vi "INI_bk9201.vi"(5 "MCListbox Ref":refnum<vi>, 9 "MCList Box Row":u8=3 max=8, 11 "Device INI Config File Path":path=path "D:/LABVIEW/Examples/INI Devices/DeviceConfig.ini") -> (0 "error out":errorcluster, 3 "Serial_VISA":T1)   [LabVIEW 2018]
uses:
  Examples - 32bit/SEQUENCER/SEQUENSER v10/Sequencer v10/Ctl/Serial_VISA.ctl
  <vilib>/Utility/miscctls.llb/LVRowAndColumnTypeDef.ctl
  <vilib>/Utility/config.llb/Read Key (String).vi
  <vilib>/Utility/config.llb/NI_LVConfig.lvlib
  <instrlib>/BK Precision 9200 Series/BK Precision 9200 Series.lvlib
panel:
  out "PowSupplay array":string[](array[string])
  out "PowSupply Read Buffer":string
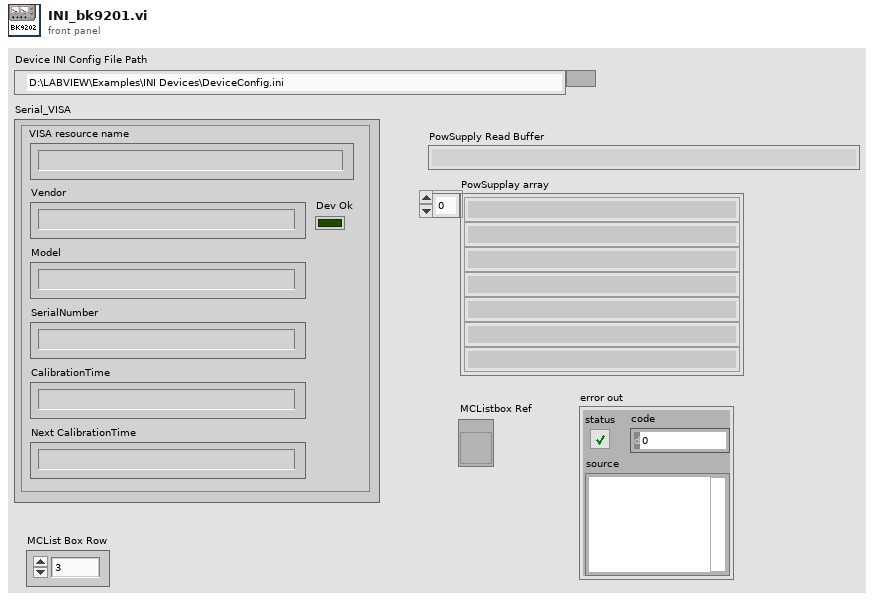
[diagram p1: front panel]
types:
  T1 = typedef "Serial_VISA.ctl" = cluster{"VISA resource name":string, "Vendor":string, "SerialNumber":string, "CalibrationTime":string, "Dev Ok":bool, "Model":string, "Next CalibrationTime":string}
  T2 = typedef "LVRowAndColumnTypeDef.ctl" = cluster{"Row":i32, "Column":i32}
  T3 = typedef "NI_LVConfig.lvlib/Config Data RefNum.ctl" = refnum<k1>
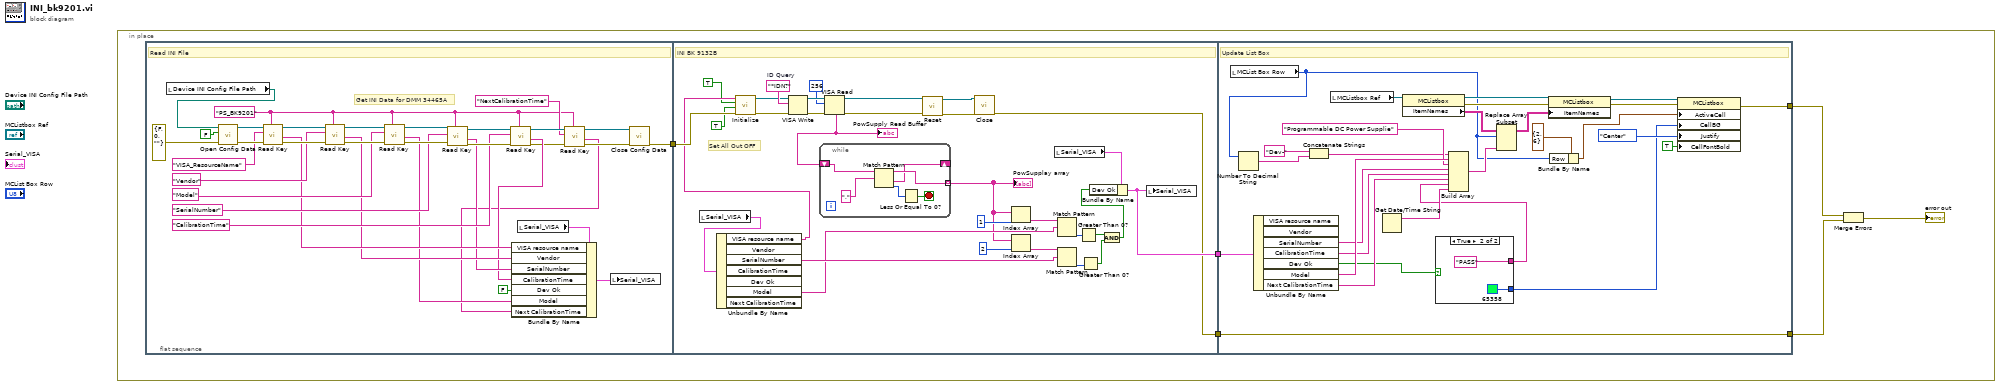
[diagram p0: block diagram]
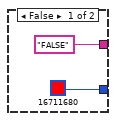
[diagram p2: hidden frame]
diagram:
  n1 = in-place {
    n2 = flat-sequence {
      tunnel: [w9] -> w6
      tunnel: w6 -> [w51]
      tunnel: [w42] -> w4
      tunnel: [w53] -> w1
      tunnel: [w85] -> w5
      tunnel: [w84] -> w3
      tunnel: w4 -> [w84]
      tunnel: w1 -> [w82]
      frame #0 {
        w13 = "PS_BK9201" ("section")
        # "Get INI Data for DMM 34465A"
        # "Read INI File"
        n3 = local read "Device INI Config File Path"() -> (w11:path)
        n4 = call <vilib>:"Open Config Data.vi"("error in (no error)"=errorcluster {"status"=FALSE, "code"=0, "source"=""} ("error constant"), "create file if necessary (T)"=FALSE, "configuration file path"=w11) -> ("error out"=w38:errorcluster, "refnum"=w39:T3)  [unwired: 6 in, 1 out]
        n5 = call-poly <vilib>:"Read Key.vi"("section"=w13, "error in (no error)"=w38, "key"="VISA_ResourceName", "refnum"=w39) -> ("error out"=w35:errorcluster, "value"=w24:string, "refnum out"=w37:T3)  [unwired: 4 in, 1 out]
        n6 = call-poly <vilib>:"Read Key.vi"("section"=w13, "error in (no error)"=w35, "key"="Vendor", "refnum"=w37) -> ("error out"=w34:errorcluster, "value"=w23:string, "refnum out"=w36:T3)  [unwired: 4 in, 1 out]
        n7 = call-poly <vilib>:"Read Key.vi"("section"=w13, "error in (no error)"=w34, "key"="Model", "refnum"=w36) -> ("error out"=w29:errorcluster, "value"=w22:string, "refnum out"=w30:T3)  [unwired: 4 in, 1 out]
        n8 = call-poly <vilib>:"Read Key.vi"("section"=w13, "error in (no error)"=w29, "key"="SerialNumber", "refnum"=w30) -> ("error out"=w26:errorcluster, "value"=w21:string, "refnum out"=w27:T3)  [unwired: 4 in, 1 out]
        n9 = call-poly <vilib>:"Read Key.vi"("section"=w13, "error in (no error)"=w26, "key"="CalibrationTime", "refnum"=w27) -> ("error out"=w17:errorcluster, "value"=w20:string, "refnum out"=w18:T3)  [unwired: 4 in, 1 out]
        n10 = local read "Serial_VISA"() -> (w8:T1)
        n11 = call-poly <vilib>:"Read Key.vi"("section"=w13, "error in (no error)"=w17, "key"="NextCalibrationTime", "refnum"=w18) -> ("error out"=w15:errorcluster, "value"=w12:string, "refnum out"=w16:T3)  [unwired: 4 in, 1 out]
        n12 = Bundle By Name(cluster=w8, "VISA resource name"=w24, "Vendor"=w23, "SerialNumber"=w21, "CalibrationTime"=w20, "Dev Ok"=FALSE, "Model"=w22, "Next CalibrationTime"=w12) -> (w7:T1)
        n13 = local write "Serial_VISA"(w7) -> ()
        n14 = call <vilib>:"Close Config Data.vi"("error in (no error)"=w15, "refnum"=w16) -> ("error out"=w9:errorcluster)  [unwired: 8 in, 1 out]
      }
      frame #1 {
        w56 = "*IDN?"  # ID Query
        # "Set All Out OFF"
        # "INI BK 9132B"
        n15 = local read "Serial_VISA"() -> (w55:T1)
        n16 = Unbundle By Name(w55) -> ("VISA resource name"=w50:string, "SerialNumber"=w66:string, "Model"=w64:string)  [unwired: 4 out]
        n17 = call <instrlib>:"Initialize.vi"("error in (no error)"=w51, "Reset (True)"=TRUE, "ID Query (True)"=TRUE, "VISA resource name"=w50) -> ("error out"=w49:errorcluster, "VISA resource name out"=w52:refnum<visa-resource-name>)  [unwired: 6 in]
        n18 = VISA Write(VISA resource name=w52, write buffer=w56, error in (no error)=w49) -> (VISA resource name out=w60:refnum<visa-resource-name>, error out=w61:errorcluster)  [unwired: 1 out]
        n19 = VISA Read(VISA resource name=w60, byte count=u32 256, error in (no error)=w61) -> (VISA resource name out=w46:refnum<visa-resource-name>, read buffer=w62:string, error out=w45:errorcluster)  [unwired: 1 out]
        "PowSupply Read Buffer" <- w62
        n20 = while {
          shift-right: [w74] -> _
          shift-left: w62 -> [w77]
          tunnel: [w75] -> w41 mode=indexing
          stop <- w72 stop-if-true
          n21 = Match Pattern(string=w77, regular expression="," ("search string/char (-)")) -> (before substring=w75:string, after substring=w74:string, offset past match=w73:i32)  [unwired: 1 in, 1 out]
          n22 = Less Or Equal To 0?(x=w73) -> (x <= 0?=w72:bool)
        }
        "PowSupplay array" <- w41
        n23 = call <instrlib>:"Reset.vi"("error in (no error)"=w45, "VISA resource name"=w46) -> ("error out"=w43:errorcluster, "VISA resource name out"=w44:refnum<visa-resource-name>)  [unwired: 8 in]
        n24 = call <instrlib>:"Close.vi"("error in (no error)"=w43, "VISA resource name"=w44) -> ("error out"=w42:errorcluster)  [unwired: 9 in]
        n25 = Index Array(array=w41, index=1) -> (element=w63:string)
        n26 = Index Array(array=w41, index=2) -> (element=w65:string)
        n27 = local read "Serial_VISA"() -> (w54:T1)
        n28 = Match Pattern(string=w63, regular expression=w64) -> (offset past match=w67:i32)  [unwired: 1 in, 3 out]
        n29 = Match Pattern(string=w65, regular expression=w66) -> (offset past match=w69:i32)  [unwired: 1 in, 3 out]
        n30 = Greater Than 0?(x=w67) -> (x > 0?=w68:bool)
        n31 = Greater Than 0?(x=w69) -> (x > 0?=w70:bool)
        n32 = And(x=w68, y=w70) -> (x .and. y?=w71:bool)
        n33 = Bundle By Name(cluster=w54, "Dev Ok"=w71) -> (w53:T1)
        n34 = local write "Serial_VISA"(w53) -> ()
      }
      frame #2 {
        # "Update List Box"
        n35 = local read "MCList Box Row"() -> (w81:u8)
        n36 = Number To Decimal String(number=w81) -> (decimal integer string=w79:string)  [unwired: 1 in]
        n37 = Unbundle By Name(w82) -> ("SerialNumber"=w102:string, "CalibrationTime"=w103:string, "Dev Ok"=w88:bool, "Model"=w104:string, "Next CalibrationTime"=w105:string)  [unwired: 2 out]
        n38 = Concatenate Strings("Dev-", w79) -> (w78:string)
        n39 = local read "MCListbox Ref"() -> (w92:refnum<vi>)
        n40 = Get Date/Time String() -> (date string=w91:string)  [unwired: 3 in, 1 out]
        n41 = property class="MCListbox"(reference=w92) -> (reference out=w95:refnum<vi>, error out=w96:errorcluster, "ItemNames"=w97:string[][])  [unwired: 1 in]
        n42 = case shown="True" w88 {
          tunnel: [u32 16711680 u32 65358] -> w87
          tunnel: ["FALSE" ("element") "PASS" ("element")] -> w86
          frame False {
          }
          frame True {
          }
        }
        n43 = Build Array(w78, w104, "Programmable DC Power Supplie", w102, w103, w105, w86, w91) -> (w99:string[])
        n44 = Replace Array Subset(array=w97, new element=w99, index (row)=w81) -> (w98:string[][])  [unwired: 1 in]
        n45 = property class="MCListbox"(reference=w95, error in=w96, "ItemNames"=w98) -> (reference out=w100:refnum<vi>, error out=w101:errorcluster)
        n46 = Bundle By Name(cluster=T2 {"Row"=2, "Column"=6} ("Active Cell:Active Cell"), "Row"=w81) -> (w89:T2)
        n47 = property class="MCListbox"(reference=w100, error in=w101, "ActiveCell"=w89, "CellBG"=w87, "Justify"=enum16{"Left", "Center", "Right"}."Center" ("Active Cell:Cell Justification"), "CellFontBold"=TRUE ("Active Cell:Cell Font:Bold")) -> (error out=w85:errorcluster)  [unwired: 1 out]
      }
    }
    n48 = Merge Errors(w5, w3) -> (→"error out":errorcluster)
  }
